vi "Phase_to_POW.vi"(1 "Phase (rad.)":dbl) -> (21 "POW":u32)   [LabVIEW 2013, in "DDS.lvlib"]
uses:
  DDS.lvlib
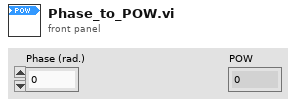
[diagram p1: front panel]
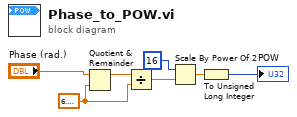
[diagram p0: block diagram]
diagram:
  w7 = 6.283185307179586
  n1 = Quotient & Remainder(x="Phase (rad.)", y=w7) -> (x-y*floor(x/y)=w4:dbl)  [unwired: 1 out]
  n2 = Divide(x=w4, y=w7) -> (x/y=w6:dbl)
  n3 = Scale By Power Of 2(n=16, x=w6) -> (x*2^n=w5:dbl)
  n4 = To Unsigned Long Integer(number=w5) -> (unsigned 32bit integer=→"POW":u32)
